vi "List Tests.vi"(8 "error in (no error)":errorcluster, 11 "LUnit Test Suite V2 in":refnum<class "LUnit Test Suite V2.lvclass">) -> (0 "error out":errorcluster, 2 "Tests":string[](array[string]), 3 "LUnit Test Suite V2 out":refnum<class "LUnit Test Suite V2.lvclass">)   [LabVIEW 2020, in "LUnit Test Suite V2.lvclass"]
uses:
  LUnit Test Suite V2.lvclass
  LUnit Test Suite V2.lvclass/LUnit Test Suite V2.ctl
  Run/Runnable.lvclass
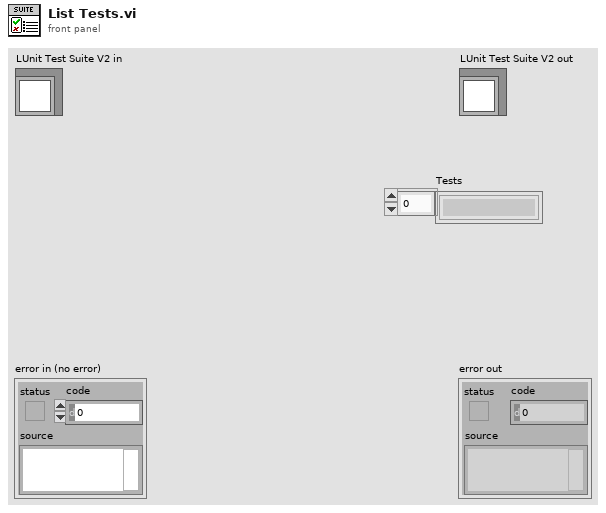
[diagram p1: front panel]
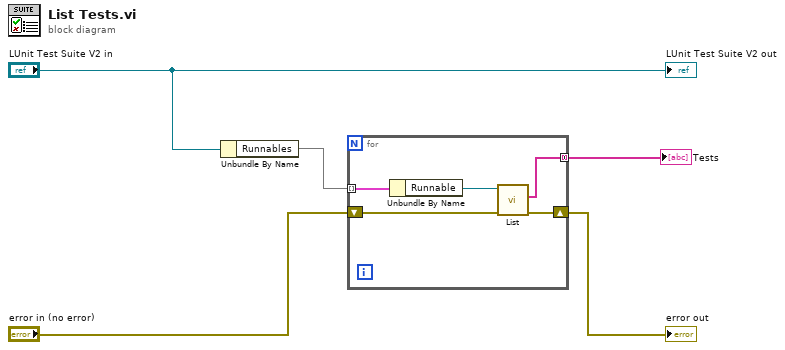
[diagram p0: block diagram]
diagram:
  n1 = Unbundle By Name("LUnit Test Suite V2 in") -> ("Runnables"=w4:map{string, refnum<class "Runnable.lvclass">})
  n2 = for {
    tunnel: w4 -> [w10] mode=indexing
    tunnel: [w8] -> w3 mode=concatenating
    shift-right: [w7] -> w2
    shift-left: "error in (no error)" -> [w6]
    n3 = Unbundle By Name(w10) -> ("Runnable"=w9:refnum<class "Runnable.lvclass">)
    n4 = call-dynamic "List.vi"("error in (no error)"=w6, "Runnable in"=w9) -> ("error out"=w7:errorcluster, "List of Runnables"=w8:string[])  [unwired: 8 in]
  }
  "error out" <- w2
  "Tests" <- w3
  "LUnit Test Suite V2 out" <- "LUnit Test Suite V2 in"
